vi "Method Quack.vi"(0 "MallardDuck in":refnum<class "MallardDuck.lvclass">, 11 "error in (no error)":errorcluster) -> (4 "MallardDuck out":refnum<class "MallardDuck.lvclass">, 15 "error out":errorcluster)   [LabVIEW 2021, in "MallardDuck.lvclass"]
uses:
  MallardDuck.lvclass
  Quacking Behaviors/Quacking Behaviors.lvclass
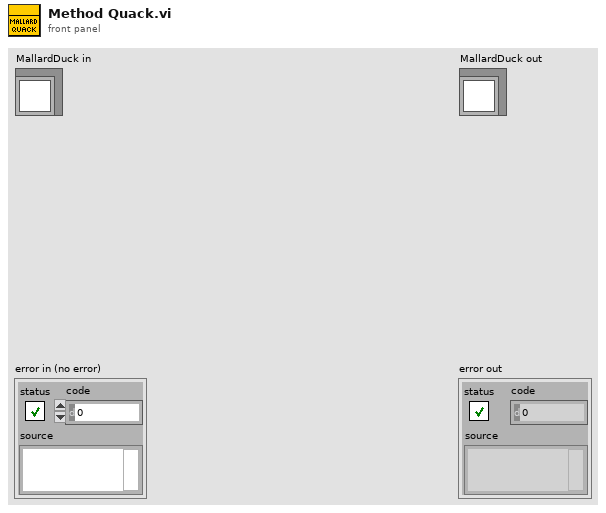
[diagram p1: front panel]
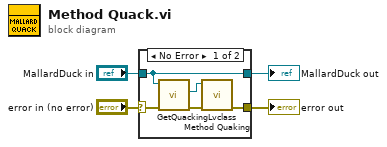
[diagram p0: block diagram]
diagram:
  n1 = case shown="No Error" "error in (no error)" {
    selector: "error in (no error)" -> [w6 w11]
    tunnel: [w9 w11] -> w3
    tunnel: "MallardDuck in" -> [w8 w10]
    tunnel: [w8 w10] -> w1
    frame No Error {
      n2 = call-dynamic "GetQuackingLvclass.vi"("error in (no error)"=w6, "object in"=w8) -> ("error out"=w5:errorcluster, "Quacking Behaviors.lvclass"=w7:refnum<class "Quacking Behaviors.lvclass">)  [unwired: 7 in, 1 out]
      n3 = call-dynamic "Method Quaking.vi"("error in (no error)"=w5, "Quacking Behaviors in"=w7) -> ("error out"=w9:errorcluster)  [unwired: 8 in, 1 out]
    }
    frame Error {
    }
  }
  "error out" <- w3
  "MallardDuck out" <- w1
